vi "Parse Driver VI Information.vi"(8 "error in (no error)":errorcluster, 10 "Version":string, 11 "CustomDeviceVI":refnum<k24>) -> (0 "error out":errorcluster, 2 "Driver VI Information":T1[](array[typedef]) {"Type" items=["Absolute", "ToBase", "ToCommonDocDir", "ToApplicationDataDir"]}, 3 "CustomDeviceVI":refnum<k24>)   [LabVIEW 2019, in "VeriStand SLSC Scripting.lvlib"]
uses:
  VeriStand SLSC Scripting.lvlib
  NationalInstruments.VeriStand.XMLReader
  Controls/Dependent File Information.ctl
  <vilib>/NI VeriStand/Custom Device API/Custom Device Supported Target.ctl
  <vilib>/NI VeriStand/Custom Device API/Custom Device API.lvlib
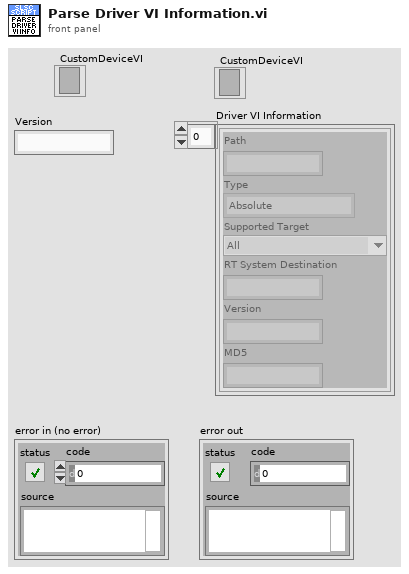
[diagram p1: front panel]
types:
  T1 = typedef "VeriStand SLSC Scripting.lvlib/Dependent File Information.ctl" = cluster{"Path":string, "Type":i32, "Supported Target":T2, "RT System Destination":string, "Version":string, "MD5":string}
  T2 = typedef "Custom Device API.lvlib/Custom Device Supported Target.ctl" = enum16{"All", "PharLap", "VxWorks", "Windows", "Linux_32_ARM", "Linux_x64", "PharLap & Windows", "PharLap & VxWorks", "VxWorks & Windows"}
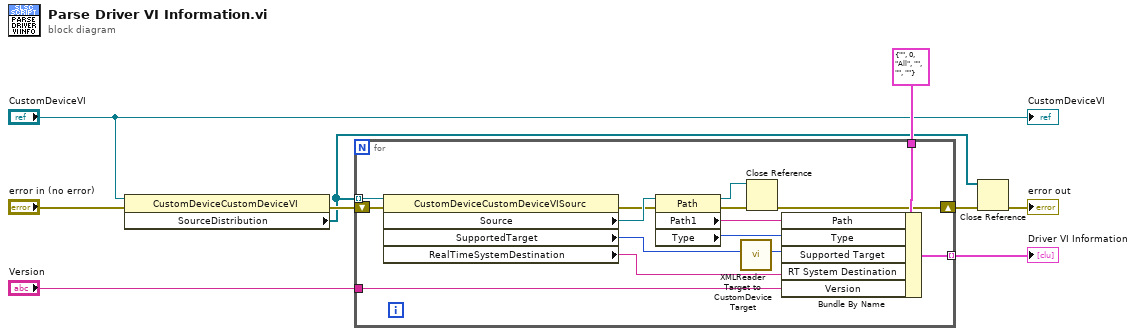
[diagram p0: block diagram]
diagram:
  n1 = property class="CustomDeviceCustomDeviceVI"(reference="CustomDeviceVI", error in="error in (no error)") -> (error out=w4:errorcluster, "SourceDistribution"=w1:refnum<k24>[])  [unwired: 1 out]
  n2 = for {
    tunnel: w1 -> [w24] mode=indexing
    tunnel: T1 {"Path"="", "Type"=0, "Supported Target"=enum."All", "RT System Destination"="", "Version"="", "MD5"=""} ("Driver VI Information") -> [w22]
    tunnel: [w18] -> w8 mode=indexing
    tunnel: "Version" -> [w17]
    shift-right: [w13] -> w9
    shift-left: w4 -> [w16]
    n3 = property class="CustomDeviceCustomDeviceVISourc"(reference=w24, error in=w16) -> (error out=w15:errorcluster, "Source"=w23:refnum<k24>, "SupportedTarget"=w11:i32, "RealTimeSystemDestination"=w19:string)  [unwired: 1 out]
    n4 = property class="Path"(reference=w23, error in=w15) -> (reference out=w12:refnum<k24>, error out=w14:errorcluster, "Path1"=w21:string, "Type"=w20:i32)
    n5 = call "XMLReader Target to CustomDevice Target.vi"("XMLReader SupportedTarget"=w11) -> ("CustomDevice Supported Target"=w10:T2)  [unwired: 10 in]
    n6 = Close Reference(reference=w12, error in (no error)=w14) -> (error out=w13:errorcluster)
    n7 = Bundle By Name(cluster=w22, "Path"=w21, "Type"=w20, "Supported Target"=w10, "RT System Destination"=w19, "Version"=w17) -> (w18:T1)
  }
  "Driver VI Information" <- w8
  n8 = Close Reference(reference=w1, error in (no error)=w9) -> (error out=→"error out":errorcluster)
  "CustomDeviceVI" <- "CustomDeviceVI"
